vi "Profile Control.vi"(6 "Control Mode":T1, 8 "error in (no error)":errorcluster, 10 "Profile Number":u32=1 min=1 step=1, 11 "Temp Chamber in":refnum<class "Temp Chamber.lvclass">) -> (0 "error out":errorcluster, 3 "Temp Chamber out":refnum<class "Temp Chamber.lvclass">)   [LabVIEW 2018, in "Temp Chamber.lvlib" / "Temp Chamber.lvclass"]
doc: "This Override is ised to Start, Pause or Stop a Profile."
uses:
  Temp Chamber.lvclass
  Custom Controls/Control Mode.ctl
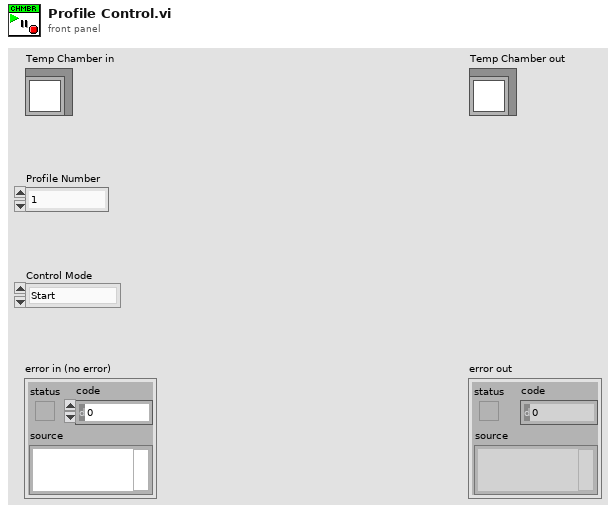
[diagram p1: front panel]
types:
  T1 = typedef "Temp Chamber.lvlib/Temp Chamber.lvclass/Control Mode.ctl" = enum16{"Start", "Pause", "Resume", "Stop"}
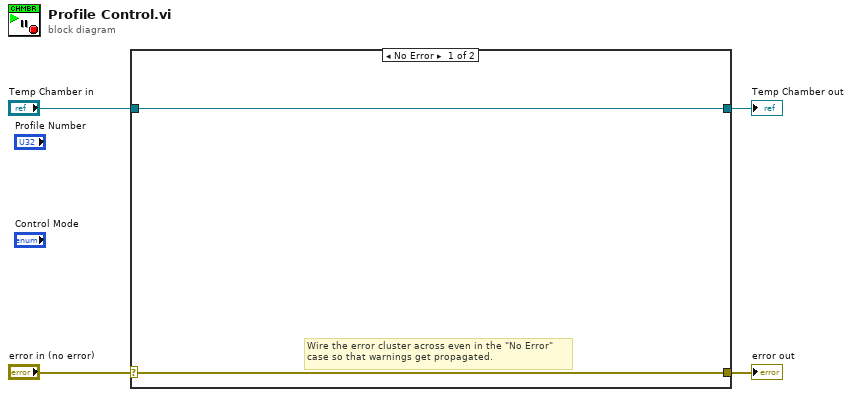
[diagram p0: block diagram]
diagram:
  n1 = case shown="No Error" "error in (no error)" {
    selector: "error in (no error)" -> [w5 w8]
    tunnel: [w5 w8] -> w3
    tunnel: [w6 w7] -> w1
    tunnel: "Temp Chamber in" -> [w6 w7]
    frame No Error {
      # "Wire the error cluster across even in the \"No Error\"\ncase so that warnings get propagated."
    }
    frame Error {
    }
  }
  "error out" <- w3
  "Temp Chamber out" <- w1
